vi "XYZ mov setup unbundler-BOOL.vi"(8 "error in (no error)":errorcluster, 9 "Keys Array":T2, 10 "Section name":string, 11 "User profile ini file ref":T1) -> (0 "error out":errorcluster, 3 "User profile ini file ref":T1)   [LabVIEW 2017]
uses:
  Typedefs/Ini file interface (Boolean).ctl
  <vilib>/Utility/config.llb/Config Data RefNum.ctl
  User Interface/Windows/Position control window/Globals/Pos ctrl window globals.vi
  <vilib>/Utility/config.llb/NI_LVConfig.lvlib
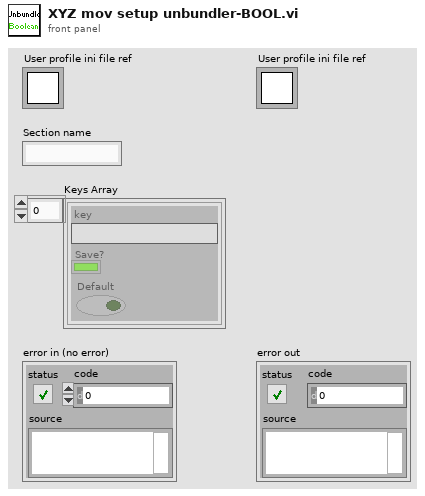
[diagram p1: front panel]
types:
  T1 = typedef "NI_LVConfig.lvlib/Config Data RefNum.ctl" = refnum<k1>
  T2 = typedef "Ini file interface (Boolean).ctl" = cluster{"key":string, "Save?":bool, "Default":bool}[]
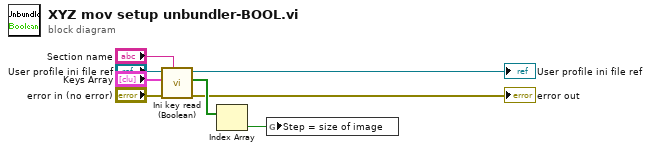
[diagram p0: block diagram]
diagram:
  n1 = call "Ini key read (Boolean).vi"("Section"="Section name", "error in (no error)"="error in (no error)", "Parameter names & setup"="Keys Array", "Ini file refnum in"="User profile ini file ref") -> ("error out"=→"error out":errorcluster, "Value read/used"=w8:bool[], "Ini file refnum out"=→"User profile ini file ref":T1)  [unwired: 5 in]
  n2 = Index Array(array=w8) -> (element=w1:bool)  [unwired: 1 in]
  n3 = global write "Pos ctrl window globals.vi" "Step = size of image"(w1) -> ()
